vi "Write Queen_.vi"(8 "error in (no error)":errorcluster, 10 "Queen?":bool=TRUE, 11 "Mother in":refnum<class "Mother.lvclass">) -> (0 "error out":errorcluster, 3 "Mother out":refnum<class "Mother.lvclass">)   [LabVIEW 2014, in "Mother.lvclass"]
uses:
  Mother.lvclass
  Mother.lvclass/Mother.ctl
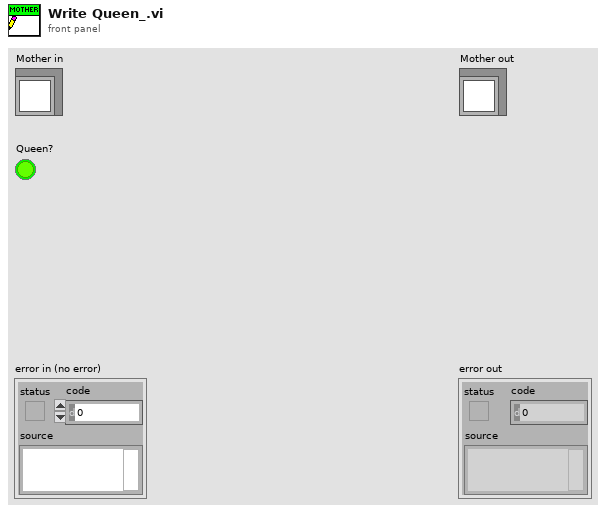
[diagram p1: front panel]
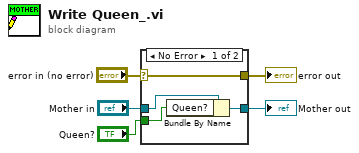
[diagram p0: block diagram]
diagram:
  n1 = case shown="No Error" "error in (no error)" {
    selector: "error in (no error)" -> [w9 w10]
    tunnel: [w9 w10] -> w4
    tunnel: [w7 w11] -> w2
    tunnel: "Mother in" -> [w8 w11]
    tunnel: "Queen?" -> [w6 _]
    frame No Error {
      n2 = Bundle By Name(cluster=w8, "Queen?"=w6) -> (w7:refnum<class "Mother.lvclass">)
    }
    frame Error {
    }
  }
  "error out" <- w4
  "Mother out" <- w2
